vi "FestoCPX.Station.Laser.Trigger.vi"(8 "error in":errorcluster, 9 "Wait (T)":bool=TRUE, 10 "Trigger":bool) -> (0 "error out":errorcluster, 2 "Aborted":bool)   [LabVIEW 2016]
uses:
  FestoCPX.DO.Signal.ctl
  tools/EventLog/EventLog.EventSource.ctl
  tools/Translator/Translator.Message.ctl
  V7310/V7310.Data.Status.State.ctl
  V7310/LowLevel/V7310.LaserStatus.ctl
  FestoCPX.DO.Data.State.Set.vi
  V7310/LowLevel/V7310.Global.vi
  tools/EventLog/EventLog.CreateError(single).vi
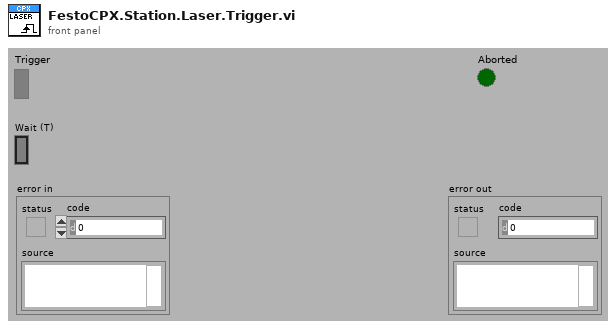
[diagram p1: front panel]
types:
  T1 = typedef "FestoCPX.DO.Signal.ctl" = enum16{"Safety Reset", "Air Main Valve", "Door Lock", "Button LED Start", "Button LED Stop", "Button LED Control", "Traffic LED Red", "Traffic LED Orange", "Traffic LED Green", "Horn", "Laser Interlock", "Laser Trigger", "Laser Fume Extractor", "Product Suction Gripper Slot 1 A", "Product Suction Gripper Slot 1 B", "Product Suction Gripper Slot 2 A", "Product Suction Gripper Slot 2 B", "Product Suction Gripper Slot 3 A", "Product Suction Gripper Slot 3 B", "Product Suction Gripper Slot 4 A", "Product Suction Gripper Slot 4 B", "Product Suction Gripper Final A", "Product Suction Gripper Final B", "Lamp", "Q1 Product Move Work", "Q1 Product Move Home", "Q2 Table Turn Work", "Q2 Table Turn Home", "Q3 Product Lift A", "Q3 Product Lift B", "Q4 Product Arm OK", "Q4 Product Arm NOK", "Q5 Product Arm Work", "Q6 Product BlowOut A", "Q6 Product BlowOut B"}
  T2 = typedef "V7310.Data.Status.State.ctl" = enum16{"First", "Init", "Msg", "Error", "Abort", "Idle", "Run"}
  T3 = typedef "Translator.Message.ctl" = enum16{"-", "Event confirmed", "Log out", "Log in", "Shutdown", "Cancel", "Start", "Begin time", "End time", "Duration", "Service Mode", "Ignore Results", "Serial Format", "On", "Off", "OK", "NOK", "NOK %s", "Home", "Work", "Close", "Open", "In progress...", "Missing", "Empty", "Hardware failure", "Initial", "Default", "Total", "Out of range", "Free disk space is below 1GB - contact technician", "Error %d >> %s", "Error %d >> %s >> %s", "Msg %d >> %s", "Laser msg %d %s", "Laser cmd error %s %d", "Laser cmd failed %s", "Laser cmd warning %s", "Laser disconnected", "Laser status %s", "Laser already started", "Laser job unkonwn %s", "Laser job missing %s", "Laser job select failure %s", "Unable to start laser printing (%s)", "Unable to stop laser printing (%s)", "Laser marking aborted", "Laser marking timeout", "Unable to reset Laser Interlock (%s)", "Unable to trigger Laser. Laser not ready (%s)", "Laser job '%s' coordinates not configured", "Starting %s", "Quitting %s", "Configured", "Initializing", "Quitting", "Loading", "Loaded %d results", "Loaded %d events", "Running", "Stopped", "Summary", "Laser", "Do you want to continue?", "Do you want to delete the configuration?", "The configuration is being used by an order. Unable to delete!", "Press confirm button", "Station is not based. Do you want to exit?", "Station requires changeover. Do you want to run the test?", "Test options are not set as default. Do you want to continue?", "Formatting of WabcoNo is disabled. Do you want to continue?", "Product not detected. Do you want to continue?", "Product scan failed. Do you want to continue?", "Calibration", "Log out?", "System", "All", "IDLE", "Translating...%s", "Not found", "Alarm %s", "Run", "Skip", "Abort", "Repeat", "Please wait...", "Database disconnected", "Database disconnected - changeover disabled!", "Login to database successful", "Login to database failed: %d; %s", "Unable to check the product status of reference %d - database disconnected", "Unable to set the product status of reference %d - database disconnected", "Variant file backup %s", "Read variant (%s)", "Result", "Station armed!", "Station requires changeover!", "Select reference number...", "EMERGENCY BUTTON - press Control button", "EMERGENCY DOOR - press Control button", "Resetting Emergency...", "Unable to reset safety circuit - Emergency Button pressed", "Unable to reset safety circuit - Emergency Side Door open", "Station not based", "Station based", "Station not empty", "Station basing...", "No order", "Press Start to begin new order", "Scanning new order", "Order NOK. Correct or scan again", "Order OK. Press Accept", "Order ready", "Revolver incorrect", "Fork incorrect", "Revolver missing", "Revolver empty", "Container missing", "Offline results", "Offline statistics", "Updating statistics %.1f %%", "DMC Configurator", "Door open", "Close the front door", "Press start button", "Done. Open the front door", "Running...", "Running...%.1f %%", "Pause %s", "Pause %s. NOK container missing", "Pause %s. OK container missing", "Pause %s. Revolver empty", "Pause %s. Revolver missing", "Pause %s. Revolver incorrect", "Pause %s. Fork missing", "Pause %s. Fork incorrect", "Pause %s. Too many failures", "Pause %s. Unloading failure", "Pause %s. One slot is not working", "Pause %s. Part order is done. Empty OK container", "Pause %s. Unable to move product to slot", "Pause %s. Unable to move back product pusher", "Pause %s. Unable to lift product", "Pause %s. Unable to move back product lifter", "Pause %s. Unable to move product arm to Work", "Pause %s. Unable to move product arm to NOK", "Pause %s. Unable to move product arm to OK", "Pause %s. Unable to unsuck the NOK product", "Pause %s. Unable to drop the NOK product", "Pause %s. Product OK missing", "Pause %s. Unable to unsuck the OK product", "Pause %s. Unable to drop the OK product", "Stopping...", "File '%s' is missing", "File '%s' is broken", "File '%s' is running", "Log file started (%s)", "Log file ended (%s)", "Log file stopped (%s)", "Log file ignored (%s)", "Log file exported (%s)", "Log file export failed (%s)", "Wrong serial number in log file", "Wrong reference number in log file", "Test steps are missing", "%s = %.3f", "Process param '%s' not found in DB", "Process param '%s' wrong order", "Process param '%s' value %.3f out of limits (%.3f; %.3f)", "Step%d param '%s' not found in DB", "Step%d param '%s' wrong order", "Step%d param '%s' value %.3f out of limits (%.3f; %.3f)", "Step%d EV '%s' not found in DB", "Step%d EV '%s' wrong order", "\"%s\" not found in DB", "\"%s\" wrong order", "\"%s\" value %.3f out of limits (%.3f; %.3f)", "\"%s\" not found in software", "Process init (%s)", "Process started", "Process restarted", "Process run", "Process done", "Process done - remove OK container", "Process aborted", "Process aborted at work", "Process aborted at home", "Process error", "Process error at home", "Process error at work", "Process close", "Process pause", "Process continue", "Process door open", "Process door close", "Process pause at slot %s due to %s", "Select plate from the order to process", "Do you want to start the process?", "Do you want to continue the process?", "There is unfinished order. Do you want to put the new order?", "Product %s %d OK", "Product %s %d NOK", "Unable to unload the slot %s. Product missing in the slot", "Unable to unload the slot %s. Product already in the arm", "Unable to accept the product as OK. Product missing in slot %s", "Unable to accept the product as OK. Product could not drop into the container at slot %s", "Unable to accept the product as NOK. Product could not drop into the container at slot %s", "Scan failed. Error %s", "Scan failed. Scanner disconnected", "Scan failed. Wrong Wabco number %d, limit (%d,%d)", "Scan failed. Wrong serial number %d, limit (%d,%d)", "Scan failed. Wrong date %d, limit (%d,%d)", "Scan failed. Wrong product wabco number %d (expected %d)", "Scan failed. Wrong product serial number %d (expected > 0)", "Scan OK %s", "Scan failed. Unable to determine table position (%s)", "Scan failed. Timeout", "Tune failed. Scanner disconnected", "Tune failed. Timeout", "%s = %d", "%s = %d->%d", "Unable to set %s = %.2f - Air Pressure Inside off", "Unable to set digital output '%s' = %d", "Unable to activate air pressure inside - timeout", "Unable to activate air pressure inside - aborted", "Unable to switch on Air Main Valve - Air Pressure Inlet off", "Unable to switch on Air Main Valve - Door open", "Unable to switch off Air Main Valve - timeout", "Unable to switch off Air Main Valve - aborted", "Unable to rotate Table - timeout", "Unable to rotate Table - aborted", "Unable to rotate Table - Product Move not in Home position", "Unable to rotate Table - Air Pressure Inside off", "Unable to rotate Table - Product Lift A not in Home position", "Unable to rotate Table - Product Lift B not in Home position", "Unable to rotate Table - unlock before movement timeout", "Unable to rotate Table - lock after movement timeout", "Unable to move Table Lock to %s position - timeout", "Unable to move Table Lock to %s position - aborted", "Unable to move Table Lock to %s position - Air Pressure Inside off", "Unable to move Table Lock to %s position - Table not in position", "Unable to move Product Lift A to %s position - timeout", "Unable to move Product Lift B to %s position - timeout", "Unable to move Product Lift A to %s position - aborted", "Unable to move Product Lift B to %s position - aborted", "Unable to move Product Lift A to %s position - Air Pressure Inside off", "Unable to move Product Lift B to %s position - Air Pressure Inside off", "Unable to move Product Lift A to %s position - Table not locked", "Unable to move Product Lift B to %s position - Table not locked", "Unable to move Product Lift A to %s position - Product Arm not in Work position", "Unable to move Product Lift B to %s position - Product Arm not in Work position", "Unable to set Product Suction Gripper %s to %s - timeout", "Unable to set Product Suction Gripper %s to %s - aborted", "Unable to set Product Suction Gripper %s to %s - Air Pressure Inside off", "Unable to set Product Suction Gripper %s to %s - Table slot unkown", "Unable to move Product Arm to %s position - timeout", "Unable to move Product Arm to %s position - aborted", "Unable to move Product Arm to %s position - Air Pressure Inside off", "Unable to move Product Arm to %s position - Product Lift A not in Home position", "Unable to move Product Arm to %s position - Product Lift B not in Home position", "Unable to move Product to %s position - timeout", "Unable to move Product to %s position - aborted", "Unable to move Product to %s position - Air Pressure Inside off", "Unable to move Product to %s position - Table not in position"}
  T4 = typedef "EventLog.EventSource.ctl" = enum16{"All", "Gui", "Ref", "File", "Arch", "Seq", "CPX", "DB", "Laser", "Scan.P", "Scan.O"}
  T5 = typedef "V7310.LaserStatus.ctl" = enum16{"-", "FatalError", "Initialize", "KeySwitchOpen", "TimeoutInterlock", "InterlockOpen", "StartUp", "ShutterlockOpen", "Standby", "Ready", "PrepareForMarking", "WaitForTrigger", "Marking"}
  T6 = typedef "V7310.Data.Status.ctl" = cluster{"State":T2, "LaserStatus":T5, "LaserStatusRaw":string, "Ref":refnum<k5>, "RTC TS":timestamp, "Conn TS":timestamp, "Msg":T7[], "JobInUse":string, "Jobs":string[], "Vars":T8[]}
  T7 = typedef "V7310.Message.Data.ctl" = cluster{"ID":i32, "Msg":string}
  T8 = typedef "V7310.Job.Variable.ctl" = cluster{"Name":string, "Value":string}
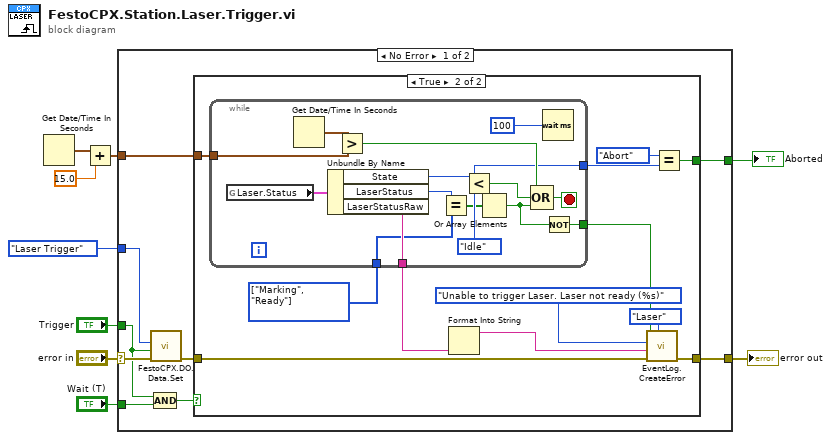
[diagram p0: block diagram]
diagram:
  n1 = Get Date/Time In Seconds() -> (seconds since 1Jan1904=w4:timestamp)
  n2 = Add(x=w4, y=15.0 ("x")) -> (x+y=w3:timestamp)
  n3 = case shown="No Error" "error in" {
    selector: "error in" -> [w18 w47]
    tunnel: [w15 w47] -> w9
    tunnel: "Trigger" -> [w13 _]
    tunnel: FestoCPX.DO.Signal."Laser Trigger" ("CPX.DO") -> [w17 _]
    tunnel: "Wait (T)" -> [w12 _]
    tunnel: w3 -> [w14 _]
    tunnel: [w10 _] -> w1
    frame No Error {
      n4 = call-poly "FestoCPX.DO.Data.Set.vi"("error in (no error)"=w18, "State"=w13, "CPX.DO"=w17) -> ("error out"=w16:errorcluster)  [unwired: 8 in]
      n5 = Compound Arithmetic op=AND(w13, w12) -> (w11:bool)
      n6 = case shown="True" w11 {
        tunnel: w16 -> [w19 w27]
        tunnel: [w19 w31] -> w15
        tunnel: w14 -> [_ w30]
        tunnel: [_ w24] -> w10
        frame False {
        }
        frame True {
          w20 = T5[] [enum."Marking", enum."Ready"] items=["-", "FatalError", "Initialize", "KeySwitchOpen", "TimeoutInterlock", "InterlockOpen", "StartUp", "ShutterlockOpen", "Standby", "Ready", "PrepareForMarking", "WaitForTrigger", "Marking"]
          n7 = while {
            tunnel: w30 -> [w43]
            tunnel: [w38] -> w29
            tunnel: [w34] -> w23
            tunnel: [w36] -> w25
            tunnel: w20 -> [w33]
            stop <- w40 stop-if-true
            n8 = global read "V7310.Global.vi" "Laser.Status"() -> (w46:T6)
            n9 = Get Date/Time In Seconds() -> (seconds since 1Jan1904=w42:timestamp)
            n10 = Unbundle By Name(w46) -> ("State"=w36:T2, "LaserStatus"=w35:T5, "LaserStatusRaw"=w34:string)
            n11 = Greater?(x=w42, y=w43) -> (0:w41:bool)
            n12 = Equal?(x=w35, y=w33) -> (x = y?=w39:bool[])
            n13 = Less?(x=w36, y=V7310.Data.Status.State."Idle" ("State")) -> (x < y?=w44:bool)
            n14 = Or Array Elements(Boolean array=w39) -> (logical OR=w32:bool)
            n15 = Compound Arithmetic op=OR(w41, w44, w32) -> (w40:bool)
            n16 = Wait (ms)(milliseconds to wait=u32 100) -> ()  [unwired: 1 out]
            n17 = Not(x=w32) -> (.not. x?=w38:bool)
          }
          n18 = Format Into String(w23) -> (resulting string=w22:string)  [unwired: 3 in, 1 out]
          n19 = call-poly "EventLog.CreateError.vi"("Source (All)"=EventLog.EventSource."Laser", "error in"=w27, "arg"=w22, "msg"=Translator.Message."Unable to trigger Laser. Laser not ready (%s)", "create (T)"=w29) -> ("error out"=w31:errorcluster)  [unwired: 6 in]
          n20 = Equal?(x=V7310.Data.Status.State."Abort", y=w25) -> (x = y?=w24:bool)
        }
      }
    }
    frame Error {
    }
  }
  "error out" <- w9
  "Aborted" <- w1
